vi "Classical Filter Design.vi"() -> ()   [LabVIEW 2023]
doc: "Demonstrates how to use the DFD Classical Design VI to design a lowpass, highpass, bandpass, or bandstop filter with classical design methods.\n\nComplete the following steps to use this VI.\n1) Run the VI.\n2) Change the specifications.\n3) Observe the magnitude response and phase response. Notice that the magnitude response approximates the frequency specification and the phase response is nonlinear for IIR filters (Butterworth, Chebyshev, Inverse Chebyshev, and Elliptic).\n4) Change the <B>Design Method</B> to view the ripples in the passband and stopband.\n5) Observe the filter order that the VI returns automatically.\n6) Click the <B>STOP</B> button to stop this VI."
uses:
  <vilib>/addons/Digital Filter Design/_Objects.llb/DFD Filter Frequence Specification (Design).ctl
  <vilib>/addons/Digital Filter Design/_Objects.llb/DFD Filter Ripple Specification (Design).ctl
  <vilib>/addons/Digital Filter Design/_Objects.llb/DFD Phase Setting.ctl
  <vilib>/addons/Digital Filter Design/Analysis.llb/DFD Plot Freq Response (Linear-Spaced).vi
  <vilib>/addons/Digital Filter Design/NI_DigFilterLicensed.lvlib
panel:
  in  "Design Method":T1(ring)=enum."Elliptic"
  in  "Filter Type":u16(ring)=2 items=["Lowpass", "Highpass", "Bandpass", "Bandstop"]
  out "Error Message":string
  in  "stop":bool
  out "Phase Response":cluster{"f0":dbl, "df":dbl, "values":dbl[]}[](graph)
  out "Magnitude Response":cluster{"f0":dbl, "df":dbl, "values":dbl[]}[](graph)
  in  "dB on?":bool=TRUE
  out "Filter Order":i32
  in  "Sampling Frequency [Hz]":dbl=1000.0 format="%.2f"
  in  "Ripple Specifications":T2={"passband"=0.1, "stopband"=60.0, "dB/linear? (T: dB)"=TRUE}
  in  "Frequency Specifications [Hz]":T3={"fpass 1"=250.0, "fstop 1"=200.0, "fpass 2 "=400.0, "fstop 2"=450.0}
  # "Select Help>>Show Context Help and move the cursor over the VI icon for more information."
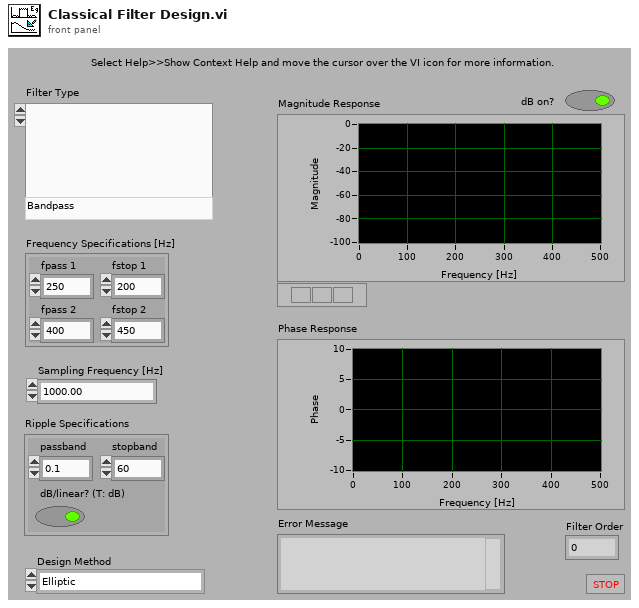
[diagram p1: front panel]
types:
  T1 = enum16{"Butterworth", "Chebyshev", "Inverse Chebyshev", "Elliptic", "Kaiser Window", "Dolph-Chebyshev Window", "Equi-Ripple FIR"}
  T2 = typedef "NI_DigFilterLicensed.lvlib/DFD Filter Ripple Specification (Design).ctl" = cluster{"passband":dbl, "stopband":dbl, "dB/linear? (T: dB)":bool}
  T3 = typedef "NI_DigFilterLicensed.lvlib/DFD Filter Frequence Specification (Design).ctl" = cluster{"fpass 1":dbl, "fstop 1":dbl, "fpass 2 ":dbl, "fstop 2":dbl}
  T4 = typedef "NI_DigFilterLicensed.lvlib/DFD Phase Setting.ctl" = cluster{"unwrap? (F)":bool, "degree? (F)":bool}
  T5 = typedef "NI_DigFilterLicensed.lvlib/DFD Filter Obj.ctl" = cluster{"mSRate_Fs":dbl, "mSRate_Version":string, "mSRate_Comments":string, "mSRate_OrgCoef":T6, "mSRate_CurCoef":T6, "mSRate_Quantized?":bool, "mSRate_QCoef":T6, "mSRate_QSettings":T8[], "mSRate_Order":i32, "mSRate_Scaling":cluster{"mSRate_ScaleByPowerOf2?":bool, "mSRate_ScaleType":T10}}
  T6 = typedef "NI_DigFilterLicensed.lvlib/DFD Filter Coef.ctl" = cluster{"type":T7, "gain":dbl, "coef a (k)":dbl[], "coef b (v)":dbl[]}
  T7 = typedef "NI_DigFilterLicensed.lvlib/DFD Filter Structure Type Selector.ctl" = enum16{"Undefined", "FIR Direct Form", "FIR Direct Form Transposed", "FIR Symmetric", "FIR Antisymmetric", "IIR Direct Form I", "IIR Direct Form I Transposed", "IIR Direct Form II", "IIR Direct Form II Transposed", "IIR Cascaded Second Order Sections Form I", "IIR Cascaded Second Order Sections Form I Transposed", "IIR Cascaded Second Order Sections Form II", "IIR Cascaded Second Order Sections Form II Transposed", "Lattice Allpass (basic sections)", "Lattice Allpass (one multiplier sections)", "Lattice Allpass (normalized sections)", "Lattice AR (basic sections)", "Lattice AR (one multiplier sections)", "Lattice AR (normalized sections)", "Lattice MA (minimum phase)", "Lattice MA (maximum phase)", "Lattice ARMA (basic sections)", "Lattice ARMA (one multiplier sections)", "Lattice ARMA (normalized sections)"}
  T8 = typedef "NI_DigFilterLicensed.lvlib/dfd_Internal Quantization Settings.ctl" = cluster{"source":T9, "wl":i16, "iwl":i16, "overflow mode":enum16{"Saturation", "Wrap"}, "rounding mode":enum16{"Nearest", "Truncation"}, "signed?":bool}
  T9 = typedef "NI_DigFilterLicensed.lvlib/dfd_Internal Quantization Srcs.ctl" = u16
  T10 = typedef "NI_DigFilterLicensed.lvlib/DFD Coef Norm Type.ctl" = enum16{"No Norm", "Time Domain 1-Norm", "Time Domain 2-Norm", "Time Domain Inf-Norm"}
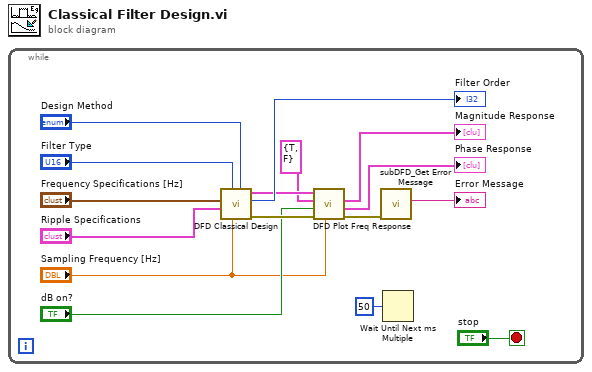
[diagram p0: block diagram]
diagram:
  n1 = while {
    stop <- "stop" stop-if-true
    n2 = call <vilib>:"DFD Classical Design.vi"("design method"="Design Method", "fs [Hz]"="Sampling Frequency [Hz]", "filter type"="Filter Type", "ripple specs"="Ripple Specifications", "freq specs [Hz]"="Frequency Specifications [Hz]") -> ("error out"=w12:errorcluster, "order"=→"Filter Order":i32, "filter out"=w13:T5)  [unwired: 1 in, 3 out]
    n3 = call-poly <vilib>:"DFD Plot Freq Response.vi"("fs [Hz]"="Sampling Frequency [Hz]", "error in (no error)"=w12, "dB on? (T)"="dB on?", "phase view"=T4 {"unwrap? (F)"=TRUE, "degree? (F)"=FALSE}, "filter in"=w13) -> ("error out"=w2:errorcluster, "phase response"=→"Phase Response":cluster{"f0":dbl, "df":dbl, "values":dbl[]}[], "magnitude response"=→"Magnitude Response":cluster{"f0":dbl, "df":dbl, "values":dbl[]}[])  [unwired: 3 in, 1 out]
    n4 = call <vilib>:"subDFD_Get Error Message.vi"("error in (no error)"=w2) -> ("Error Message"=→"Error Message":string)  [unwired: 10 out]
    n5 = Wait Until Next ms Multiple(millisecond multiple=u32 50) -> ()  [unwired: 1 out]
  }
